vi "Limit to available tests.vi"(8 "error in (no error)":errorcluster, 11 "Test Selector in":refnum<class "Test Selector.lvclass">) -> (0 "error out":errorcluster, 3 "Test Selector out":refnum<class "Test Selector.lvclass">)   [LabVIEW 2019, in "Test Selector.lvlib" / "Test Selector.lvclass"]
uses:
  Test Selector.lvclass
  Test Selector.lvclass/Test Selector.ctl
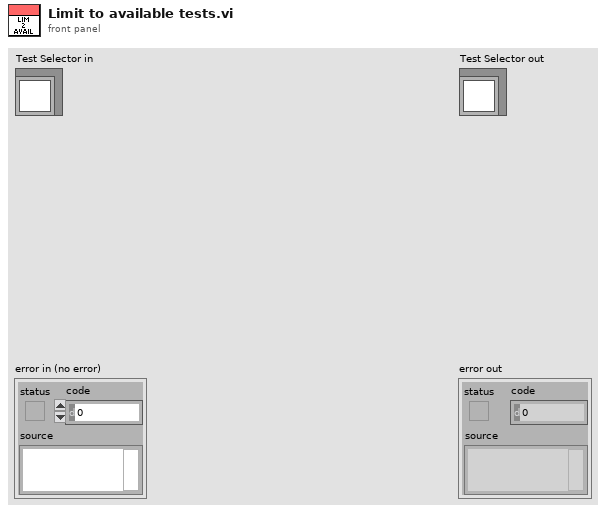
[diagram p1: front panel]
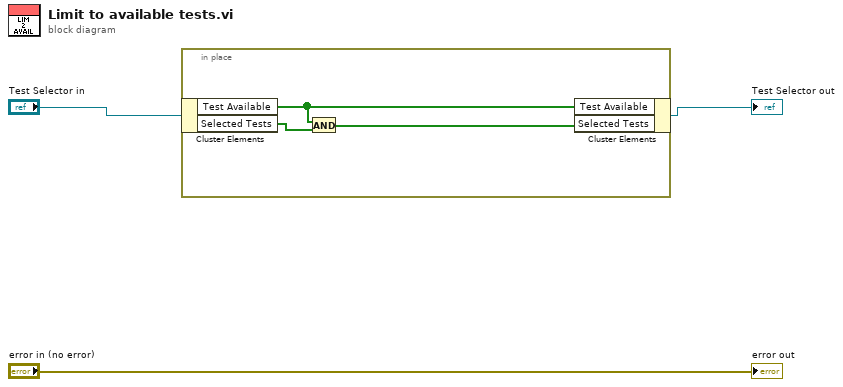
[diagram p0: block diagram]
diagram:
  n1 = in-place {
    n2 = in-place-cluster #1("Test Selector in") -> ("Test Available"=w5:bool[], "Selected Tests"=w6:bool[])
    n3 = And(x=w5, y=w6) -> (x .and. y?=w4:bool[])
    n4 = in-place-cluster #1("Test Available"=w5, "Selected Tests"=w4) -> (→"Test Selector out":refnum<class "Test Selector.lvclass">)
  }
  "error out" <- "error in (no error)"
